vi "getWavelength_v80AM4.vi"() -> ()   [LabVIEW 2016]
uses:
  <vilib>/Analysis/baseanly.llb/Mean (DBL).vi
  x32/CLDevIFace.dll
  <vilib>/Analysis/NI_AALBase.lvlib
panel:
  in  "Avg":i32=1
  out "Delta MHz":dbl
  in  "Scale Factor":dbl=800.0
  out "Power (mW)":dbl format="%.9f"
  out "return type":i32
  in  "Clear Chart?":bool
  in  "Delay Time (s)":dbl=0.01
  out "XY Graph":cluster{i32[], dbl[]}(graph)
  out "error out":errorcluster
  out "output param":i32
  in  "stop":bool
  in  "OK Button":bool
  out "Wavelength":dbl format="%.9f"
  in  "CommPort":dbl=5.0 caption="Comm Port #"
  # "Super cavity FSR  6 GHz\nZerodure FSR  750 MHz"
  # "1 pm = 200 MHz @1212nm\n1 pm = 800 MHz @606 nm"
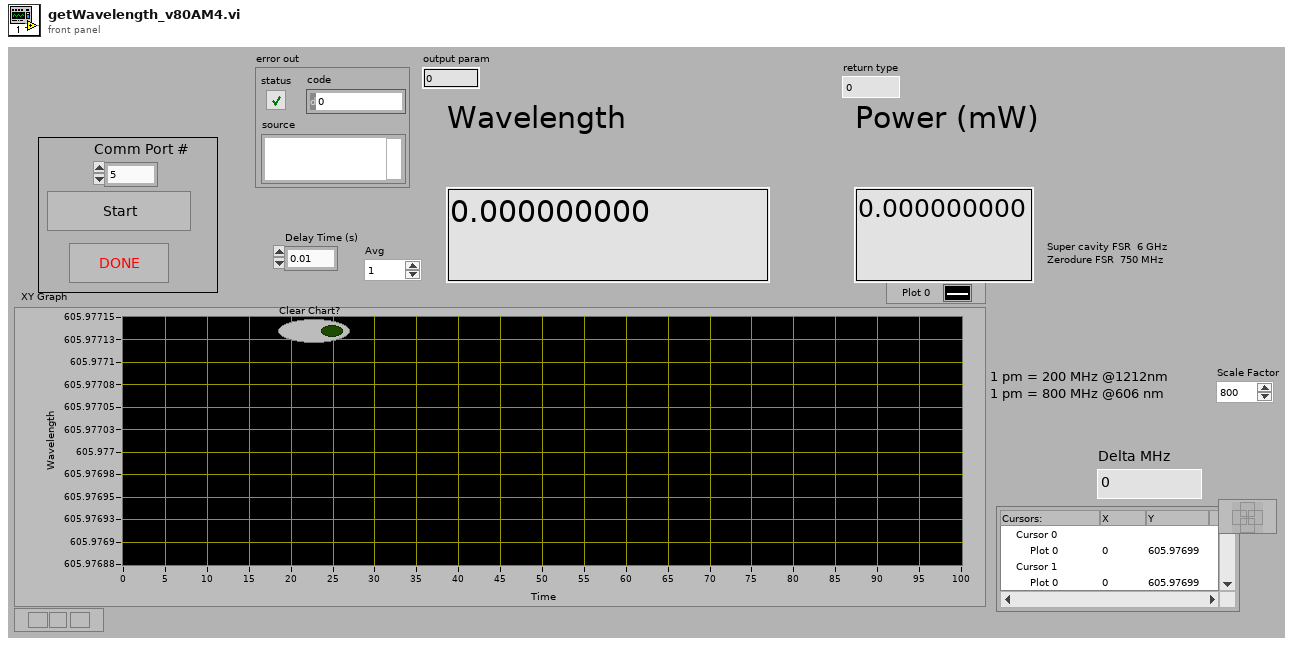
[diagram p1: front panel]
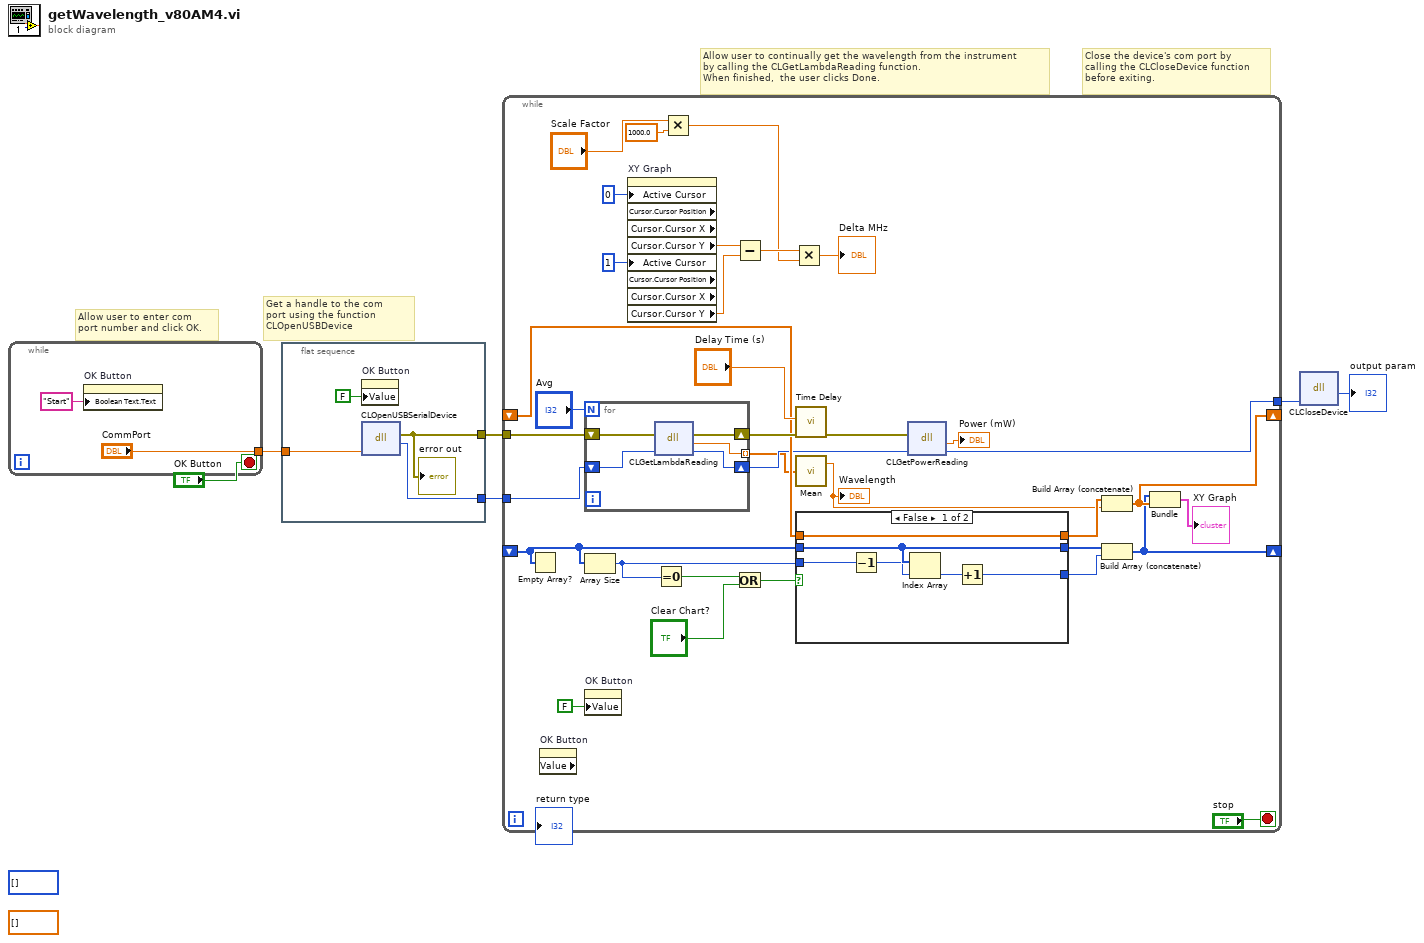
[diagram p0: block diagram]
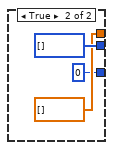
[diagram p2: hidden frame]
diagram:
  (unwired) i32[] []
  (unwired) dbl[] []
  # "Close the device's com port by\ncalling the CLCloseDevice function\nbefore exiting."
  # "Allow user to continually get the wavelength from the instrument\nby calling the CLGetLambdaReading function.  \nWhen finished,  the user clicks Done."
  # "Get a handle to the com\nport using the function CLOpenUSBDevice"
  # "Allow user to enter com \nport number and click OK."
  n1 = while {
    tunnel: ["CommPort"] -> w5
    stop <- "OK Button" stop-if-true
    n2 = property on="OK Button" class="Bool (strict)"("Boolean Text.Text"="Start") -> ()  [unwired: 2 in, 2 out]
  }
  n3 = flat-sequence {
    tunnel: w5 -> [w12]
    tunnel: [w11] -> w4
    tunnel: [w9] -> w1
    frame #0 {
      n4 = property on="OK Button" class="Bool (strict)"("Value"=FALSE) -> ()  [unwired: 2 in, 2 out]
      n5 = dll-call lib="C:/Users/Lab/Desktop/Bristol wavemeter 621/00424-2-00 621 customer CD/Programming Interface/x32/CLDevIface.dll" fn="CLOpenUSBSerialDevice"("commPort"=w12) -> (error out=w9:errorcluster, "return type"=w11:i32)  [unwired: 4 in, 1 out]
      "error out" <- w9
    }
  }
  n6 = while {
    tunnel: w4 -> [w46]
    tunnel: [w33] -> w3
    shift-right: [w43] -> _
    shift-left: _ -> [w37]
    shift-right: [w42] -> _
    shift-left: _ -> [w18]
    tunnel: w1 -> [w38]
    stop <- "stop" stop-if-true
    n7 = Empty Array?(array=w18) -> ()  [unwired: 1 out]
    n8 = property on="OK Button" class="Bool (strict)" props=["Value"]() -> ()  [unwired: 2 in, 3 out]
    n9 = for {
      N: "Avg" -> [_]
      tunnel: [w50] -> w16 mode=indexing
      shift-right: [w47] -> w34
      shift-left: w46 -> [w51]
      shift-right: [w49] -> w39
      shift-left: w38 -> [w48]
      n10 = dll-call lib="C:/Users/Lab/Desktop/Bristol wavemeter 621/00424-2-00 621 customer CD/Programming Interface/x32/CLDevIface.dll" fn="CLGetLambdaReading"(error in=w48, "devHandle"=w51) -> (error out=w49:errorcluster, "return type"=w50:dbl, "devHandle"=w47:i32)  [unwired: 2 in, 1 out]
    }
    n11 = Array Size(array=w18) -> (size(s)=w14:i32)
    n12 = property on="OK Button" class="Bool (strict)"("Value"=FALSE) -> ()  [unwired: 2 in, 2 out]
    n13 = property on="XY Graph" class="XYGraph (strict)" props=["Active Cursor", "Cursor", "Cursor Position", "Cursor", "Cursor X", "Cursor", "Cursor Y", "Active Cursor", "Cursor", "Cursor Position", "Cursor", "Cursor X", "Cursor", "Cursor Y"]("Active Cursor"=u32 0, "Active Cursor"=u32 1) -> ("Cursor.Cursor Y"=w29:dbl, "Cursor.Cursor Y"=w30:dbl)  [unwired: 2 in, 6 out]
    n14 = Equal To 0?(x=w14) -> (x = 0?=w23:bool)
    n15 = Multiply(x="Scale Factor", y=1000.0) -> (x*y=w24:dbl)
    n16 = Subtract(x=w29, y=w30) -> (x-y=w31:dbl)
    n17 = Or(x=w23, y="Clear Chart?") -> (x .or. y?=w21:bool)
    n18 = Multiply(x=w31, y=w24) -> (x*y=→"Delta MHz":dbl)
    n19 = call "Time Delay"("error in (no error)"=w39, "Delay Time (s)"="Delay Time (s)") -> ("error out"=w36:errorcluster)  [unwired: 9 in]
    n20 = call-poly <vilib>:"Mean.vi"("X"=w16) -> ("mean"=w15:dbl)  [unwired: 1 out]
    "Wavelength" <- w15
    n21 = case shown="False" w21 {
      tunnel: w37 -> [w57 _]
      tunnel: w18 -> [w56 _]
      tunnel: [w56 i32[] []] -> w19
      tunnel: [w57 dbl[] []] -> w20
      tunnel: w14 -> [w53 _]
      tunnel: [w54 0] -> w13
      frame False {
        n22 = Decrement(x=w53) -> (x-1=w52:i32)
        n23 = Index Array(array=w56, index=w52) -> (element=w55:i32)
        n24 = Increment(x=w55) -> (x+1=w54:i32)
      }
      frame True {
      }
    }
    n25 = dll-call lib="C:/Users/Lab/Desktop/Bristol wavemeter 621/00424-2-00 621 customer CD/Programming Interface/x32/CLDevIface.dll" fn="CLGetPowerReading"(error in=w36, "devHandle"=w34) -> ("return type"=→"Power (mW)":dbl, "devHandle"=w33:i32)  [unwired: 2 in, 2 out]
    n26 = Build Array (concatenate)(w20, w15) -> (w43:dbl[])
    n27 = Build Array (concatenate)(w19, w13) -> (w42:i32[])
    n28 = Bundle(w42, w43) -> (→"XY Graph":cluster{i32[], dbl[]})  [unwired: 1 in]
  }
  n29 = dll-call lib="C:/Users/Lab/Desktop/Bristol wavemeter 621/00424-2-00 621 customer CD/Programming Interface/x32/CLDevIface.dll" fn="CLCloseDevice"("commPort"=w3) -> ("return type"=→"output param":i32)  [unwired: 4 in, 2 out]
